vi "Main.vi"() -> ()   [LabVIEW 2018, in "Tracks Repair.lvlib"]
doc: "This template is based off of the Queued Message Handler design pattern and the Queued Message Handler project template that ships with LabVIEW.\n\nThe main difference is that the queue is private to this module and communication between modules is performed via Broadcast and Request events.\n\nRequest events are wrapped in public API methods and are handled in the Event Handling Loop (EHL) of this VI. Any module can register for Broadcast events sent by this module. The EHL generates messages based on user interface actions.\n\nThe Message Handling Loop (MHL) processes messages generated by the EHL, or by other messages. The messages are string values, so new messages can be added easily to the Message Cases case structure in the MHL. Each message cluster can also provide an optional value for Message Data, which is a variant that can be converted to whatever message-specific data is required.\n_____\nBased on Delacor QMH Project Template 4.2.1.64."
uses:
  Tracks Repair.lvlib
  <vilib>/Delacor/Delacor QMH/Libraries/Module Admin_class/Delacor_lib_QMH_Module Admin.lvclass
  SubVi's/Controls/CTL_Basic_cage_settings.ctl
  SubVi's/Controls/CTL_Filter_selector.ctl
  SubVi's/Controls/CTL_Cage_radial_segmentation.ctl
  Module Data--cluster.ctl
  Private API/Data.lvclass
  <vilib>/Delacor/Delacor QMH/Libraries/Message Queue_class/Delacor_lib_QMH_Message Queue.lvclass/Delacor_lib_QMH_Message Queue.ctl
  Stop Argument--cluster.ctl
  <vilib>/Delacor/Delacor QMH/Libraries/Module Admin_class/Delacor_lib_QMH_Module Admin.lvclass/Delacor_lib_QMH_Module Admin.ctl
  Private API/Arguments/Open folder Argument--cluster.ctl
  Private API/Arguments/Load filelist Argument--cluster.ctl
  Private API/Arguments/Preprocess filelist Argument--cluster.ctl
  Show list of files Argument--cluster.ctl
  Show Specific Track Argument--cluster.ctl
  <vilib>/Utility/miscctls.llb/LVPointTypeDef.ctl
  Private API/Data.lvclass/Data.ctl
  <vilib>/Utility/sysdir.llb/System Directory Type.ctl
  SubVi's/Controls/CTL_Post-processing_params.ctl
  SubVi's/Controls/CTL_Mouse_Draw_Params.ctl
  <vilib>/vision/Image Controls.llb/IMAQ Image.ctl
  SubVi's/Controls/CTL_Calibration_parameters.ctl
  SubVi's/Controls/CTL_Dispenser_calibration_info.ctl
  SubVi's/Controls/CTL_Pixel_to_Zone_array.ctl
  <vilib>/Delacor/Delacor QMH/Libraries/Message Queue_class/Delacor_lib_QMH_Enqueue Message (Single).vi
  <vilib>/Delacor/Delacor QMH/Libraries/Module Admin_class/Delacor_lib_QMH_Get External Launch.vi
  Private API/Methods/Write Status.vi
  Private API/Methods/Write Directory path.vi
  Private API/Methods/Write TDMS files paths.vi
  Private API/Methods/Read Directory path.vi
  Private API/Methods/Read TDMS files paths.vi
  <vilib>/Utility/error.llb/Error Cluster From Error Code.vi
  <userlib>/_OpenG.lib/file/file.llb/File Exists - Scalar__ogtk.vi
  <vilib>/ErrorRing/Error Ring.xnode
  <vilib>/Delacor/Delacor QMH/Libraries/Message Queue_class/Delacor_lib_QMH_Message Queue.lvclass
  Tracker.lvlib
panel:
  in  "Cage radial segmentation":T1={"CENTER"={"Radius, mm CENTER"=30}, "MIDFIELD"={"Radius, mm MIDFIELD"=75, "N segments MIDFIELD"=2, "Starting angle MIDFIELD"=0}, "BORDER"={"N segments BORDER"=4, "Starting angle BORDER"=0}} caption="Segmentation" {"BORDER"."N segments BORDER" min=1 max=12; "MIDFIELD"."N segments MIDFIELD" max=8; "CENTER"."Radius, mm CENTER" min=5 step=1}
  in  "Refresh Button":bool
  in  "Apply to All Button":bool
  in  "Apply Button":bool
  in  "Data filtering":T2={"Filter type"=enum."Savitzky-Golay", "Length"=41, "Order"=3} {"Order" min=3 max=11 step=2; "Length" min=5 max=301 step=2}
  in  "Decimate":bool=TRUE
  in  "Diagram (display)":T3(plugin-control)=refnum
  out "Rec. start (SW)":timestamp format="%<%H:%M:%S%3u %Y.%m.%d>T"
  out "Rec. start (HW)":i32
  in  "Settings":T4={"Vert. offset"=0.0, "Hor. offset"=0.0, "Bridge swap"=FALSE, "Twisted neck"=FALSE, "Cage diam."=325, "Magn.rot."=0, "Acq. speed"=0.0} {"Acq. speed" format="%_5f fps"; "Magn.rot." min=-180 max=180 step=1 format="%.0d°"; "Cage diam." format="%.0u mm"; "Hor. offset" format="%#_1f mm"; "Vert. offset" format="%#_1f mm"}
  in  "Open Button":bool
  in  "List of files":i32(listbox)
  in  "Simulate MHL Error":bool
  in  "Simulate EHL Error":bool
  out "error out":errorcluster
  in  "Module Admin":refnum<class "Delacor_lib_QMH_Module Admin.lvclass">
  out "Status":string
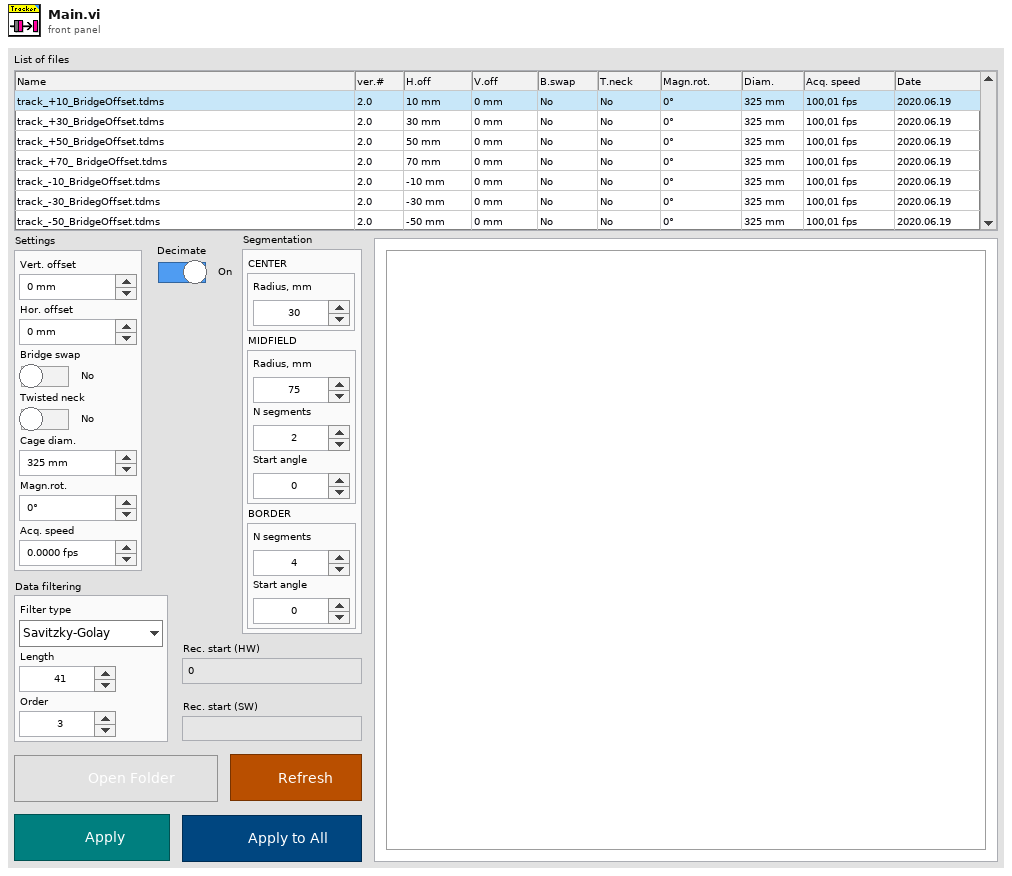
[diagram p1: front panel]
types:
  T1 = typedef "Tracker.lvlib/CTL_Cage_radial_segmentation.ctl" = cluster{"CENTER":cluster{"Radius, mm CENTER":u16}, "MIDFIELD":cluster{"Radius, mm MIDFIELD":u16, "N segments MIDFIELD":u8, "Starting angle MIDFIELD":i16}, "BORDER":cluster{"N segments BORDER":u8, "Starting angle BORDER":i16}}
  T2 = typedef "Tracker.lvlib/CTL_Filter_selector.ctl" = cluster{"Filter type":enum16{"None", "Savitzky-Golay"}, "Length":i32, "Order":i32}
  T3 = typedef "IMAQ Image.ctl" = refnum<image>
  T4 = typedef "Tracker.lvlib/CTL_Basic_cage_settings.ctl" = cluster{"Vert. offset":dbl, "Hor. offset":dbl, "Bridge swap":bool, "Twisted neck":bool, "Cage diam.":i32, "Magn.rot.":i32, "Acq. speed":dbl}
  T5 = typedef "Tracks Repair.lvlib/Module Data--cluster.ctl" = cluster{"Status":string}
  T6 = typedef "Tracks Repair.lvlib/Request Events--cluster.ctl" = cluster{"Stop Module":refnum<user-event>, "Show Panel":refnum<user-event>, "Hide Panel":refnum<user-event>, "Get Module Execution Status":refnum<user-event>, "Show Diagram":refnum<user-event>, "Open folder":refnum<user-event>, "Load filelist":refnum<user-event>, "Preprocess filelist":refnum<user-event>, "Show list of files":refnum<user-event>, "Show Specific Track":refnum<user-event>}
  T7 = enum32{"invalid lock state", "Not Locked", "Locked (No Password)", "Password-protected"}
  T8 = typedef "Tracks Repair.lvlib/Stop Argument--cluster.ctl" = cluster{"Origin":string, "Exit via Stop Module Req?":bool, "Wait for Module to stop?":bool}
  T9 = typedef "Tracks Repair.lvlib/Open folder Argument--cluster.ctl" = cluster{"Open":bool}
  T10 = typedef "Tracks Repair.lvlib/Load filelist Argument--cluster.ctl" = cluster{"Boolean":bool}
  T11 = typedef "Tracks Repair.lvlib/Preprocess filelist Argument--cluster.ctl" = cluster{"Boolean":bool}
  T12 = typedef "Tracks Repair.lvlib/Show list of files Argument--cluster.ctl" = cluster{"Boolean":bool}
  T13 = typedef "Tracks Repair.lvlib/Show Specific Track Argument--cluster.ctl" = cluster{"Track #":i32}
  T14 = typedef "LVPointTypeDef.ctl" = cluster{"Horizontal":i16, "Vertical":i16}
  T15 = enum32{"Invalid", "Standard", "Closed", "Hidden", "Minimized", "Maximized"}
  T16 = typedef "Tracker.lvlib/CTL_Post-processing_params.ctl" = cluster{"Defragment TDMS? (F)":bool, "Start time (SW)":timestamp, "Start time (HW)":u32, "Data filtering":T2, "Mouse drawing parameters":T17, "Size of the image (480x480)":cluster{"Numeric Control":dbl, "Numeric Control":dbl}, "Image ref. in":T3, "Calibration parameters":T18, "Pixel to zone":T20}
  T17 = typedef "Tracker.lvlib/CTL_Mouse_Draw_Params.ctl" = cluster{"Trace length, samples":u16, "Rainbow track":bool, "Rainbow track is speed":bool, "Bright mouse lineout":bool, "Colors array":u32[], "Pixels per mm":dbl}
  T18 = typedef "Tracker.lvlib/CTL_Calibration_parameters.ctl" = cluster{"Timing calibration sw/hw":dbl, "True FPS":dbl, "True frame time, s":dbl, "Disp. calibration info":T19}
  T19 = typedef "Tracker.lvlib/CTL_Dispenser_calibration_info.ctl" = cluster{"Channel":u8, "Speed, µl per ms":dbl}[]
  T20 = typedef "Tracker.lvlib/CTL_Pixel_to_Zone_array.ctl" = i8[][]
  T21 = typedef "System Directory Type.ctl" = i32
  T22 = typedef "Tracker.lvlib/CTL_Settings_cluster.ctl" = cluster{"Defaults":cluster{"Default User":dbl, "VISA Resource Name ":string, "Histogram parameters":T23}, "Recording and saving":cluster{"Researcher name":string, "Name prefix":string, "Data post-processing":T2, "Stop at":dbl, "\"Stop at\" enabled":bool, "Default save folder path":path, "Acquisition FPS":T24}, "Geometry":T25, "IO parameters":T26, "Conditions presets array":T27, "Calibration parameters":T18, "Settings loaded OK":bool}
  T23 = typedef "Tracker.lvlib/CTL_Histogram_parameters.ctl" = cluster{"max":dbl, "min":dbl, "# bins":i32, "threshold":dbl, "thr. type":enum16{"higher accepted", "lower accepted"}}
  T24 = typedef "Tracker.lvlib/CTL_Acquisition_speed_selector.ctl" = enum16{"Max", "Optimal", "Eco"}
  T25 = typedef "Tracker.lvlib/CTL_Segmented_plot_parameters.ctl" = cluster{"Cage diameter, mm":u16, "Starting angle MIDFIELD":i16, "Starting angle BORDER":i16, "Radius, mm CENTER":u16, "Radius, mm MIDFIELD":u16, "N segments MIDFIELD":u8, "N segments BORDER":u8, "R-gap, mm":sgl, "Bridge swap":bool, "Bridge H. offset":sgl, "Bridge V. offset":sgl, "Twisted neck":bool, "Alt. magn. orientation":bool, "Sensor board size":enum16{"Small", "Large"}}
  T26 = typedef "Tracker.lvlib/CTL_IO_params_cluster.ctl" = cluster{"IO general config.":u16, "IO 1 configuration":u16, "IO 2 configuration":u16, "IO 3 configuration":u16, "IO 4 configuration":u16, "Activate ext. RS-232":u16, "IO inversion config.":u16, "Sync capability":u8}
  T27 = typedef "Tracker.lvlib/CTL_Conditions_Array.ctl" = T28[]
  T28 = typedef "Tracker.lvlib/CTL_Conditions_Cluster.ctl" = cluster{"Enabled":bool, "Name":string, "Specifier(s)":cluster{"Specifier enabled":bool, "Condition type":T29, "Comparison type":T30, "Value":dbl, "Validity criteria(s)":cluster{"V. check enabled":bool, "Criteria":T31, "Validity value":dbl}[]}[], "Response":T32, "Has been set":bool}
  T29 = typedef "Tracker.lvlib/CTL_Condition_type.ctl" = enum16{"Speed", "Zone", "Angle to wall"}
  T30 = typedef "Tracker.lvlib/CTL_Comparison_type.ctl" = enum16{"Less", "Less or Equal", "Equal", "Greater or Equal", "Greater", "Not Equal"}
  T31 = typedef "Tracker.lvlib/CTL_Validity_check_criteria.ctl" = enum16{"Running bout (seconds)", "Running bout (meters)"}
  T32 = typedef "Tracker.lvlib/CTL_Response_info.ctl" = cluster{"Response type":T33, "TTL port":T34, "TTL pulse length, ms":dbl}
  T33 = typedef "Tracker.lvlib/CTL_Condition_response_type.ctl" = enum16{"None", "Air puff", "Liquid reward"}
  T34 = typedef "Tracker.lvlib/CTL_Reponse_port_info.ctl" = enum16{"Port 1", "Port 2", "Port 3", "Port 4"}
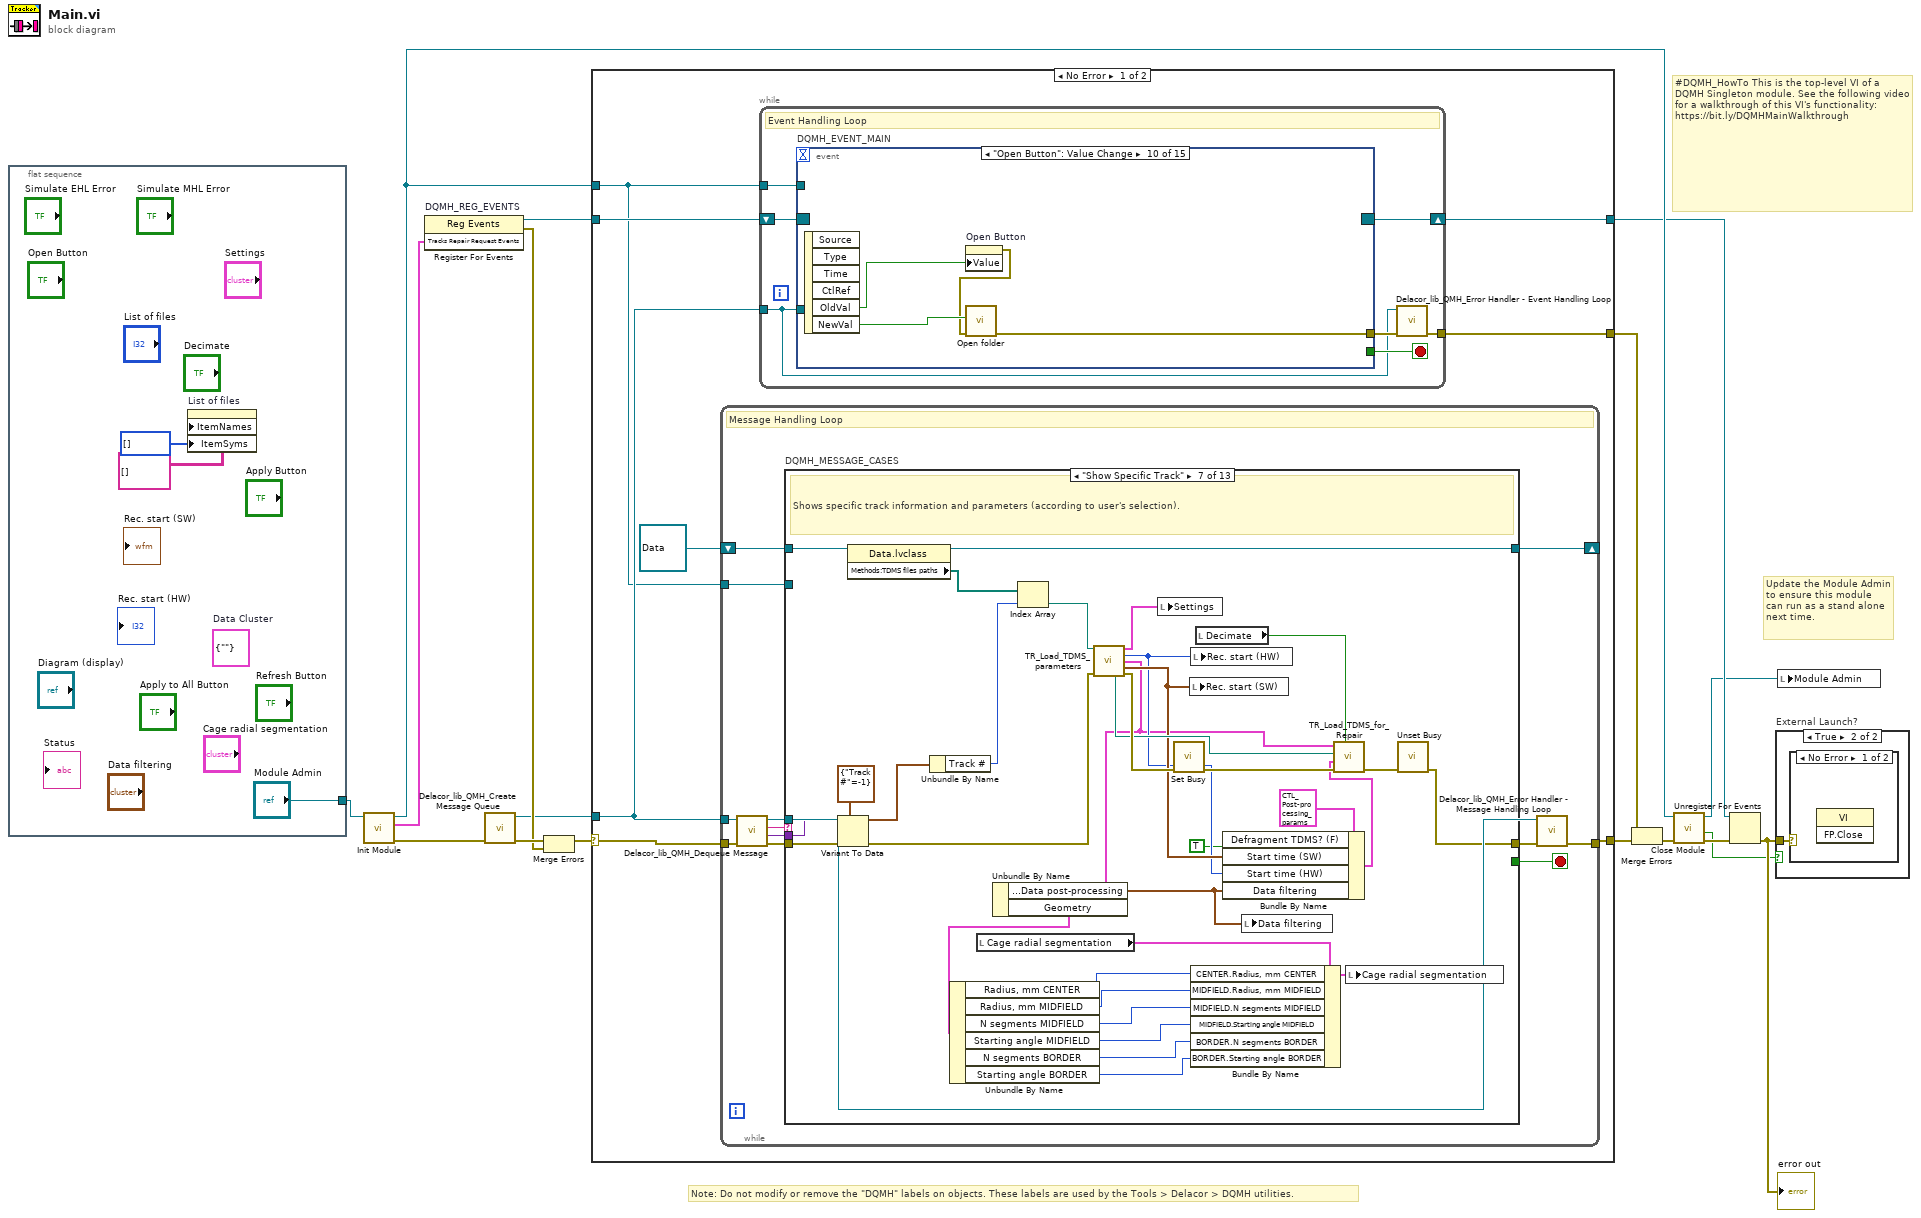
[diagram p0: block diagram]
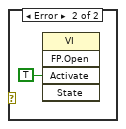
[diagram p3: hidden frame]
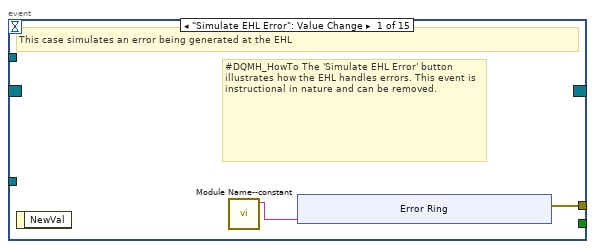
[diagram p4: hidden frame]
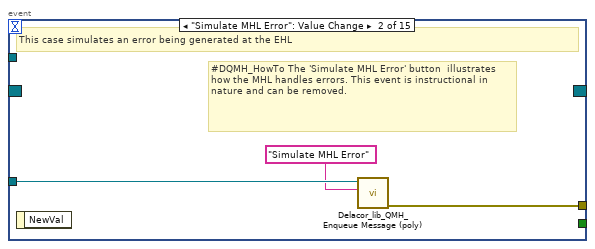
[diagram p5: hidden frame]
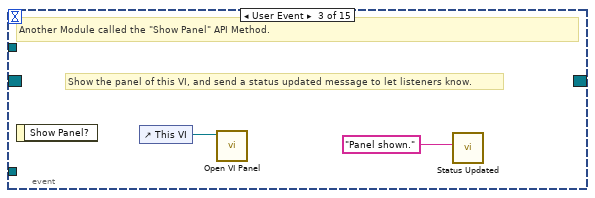
[diagram p6: hidden frame]
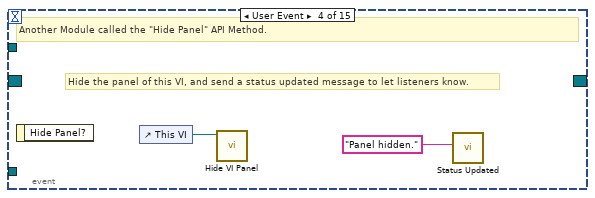
[diagram p7: hidden frame]
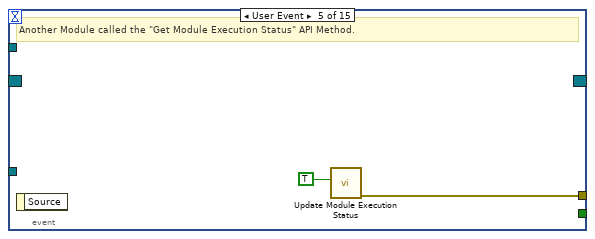
[diagram p8: hidden frame]
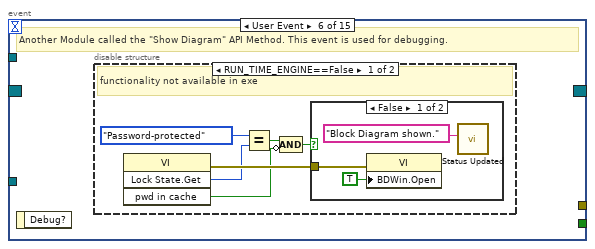
[diagram p9: hidden frame]
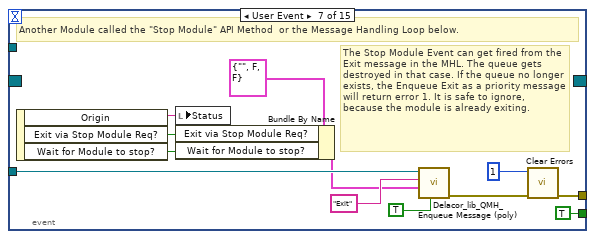
[diagram p12: hidden frame]
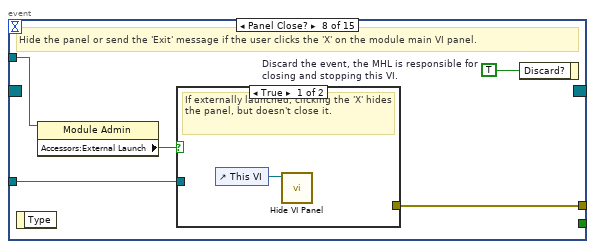
[diagram p13: hidden frame]
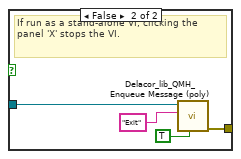
[diagram p14: hidden frame]
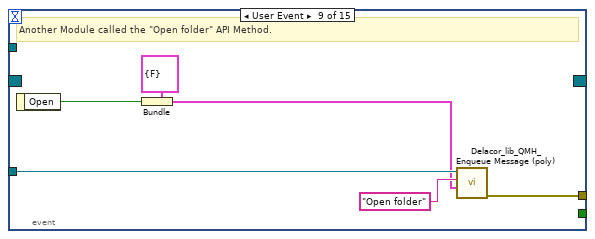
[diagram p15: hidden frame]
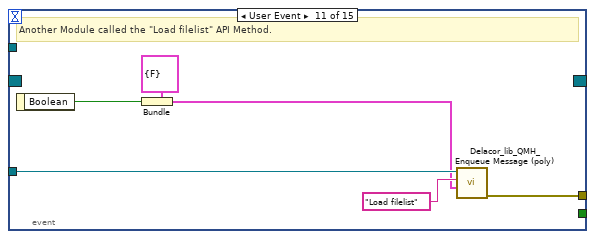
[diagram p16: hidden frame]
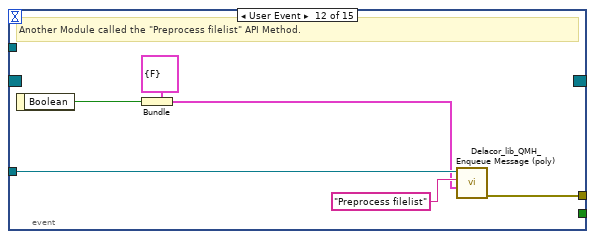
[diagram p17: hidden frame]
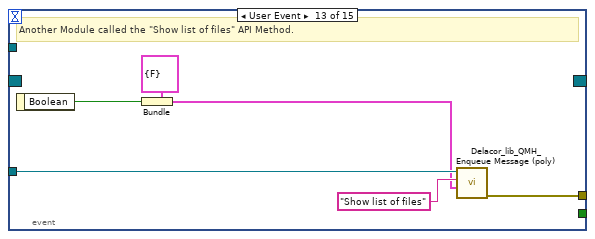
[diagram p18: hidden frame]
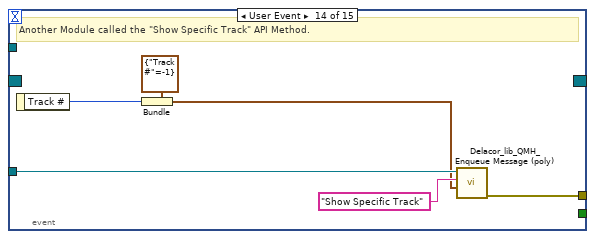
[diagram p19: hidden frame]
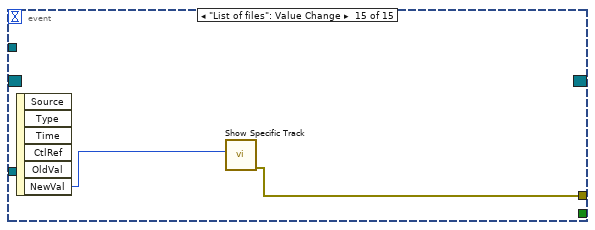
[diagram p20: hidden frame]
diagram:
  # "#DQMH_HowTo This is the top-level VI of a DQMH Singleton module. See the following video for a walkthrough of this VI's functionality: https://bit.ly/DQMHMainWalkthrough"
  # "Note: Do not modify or remove the \"DQMH\" labels on objects. These labels are used by the Tools > Delacor > DQMH utilities."
  # "Update the Module Admin to ensure this module can run as a stand alone next time."
  n1 = flat-sequence {
    tunnel: ["Module Admin"] -> w3
    frame #0 {
      (unwired) T5 {"Status"=""}  # Data Cluster
      n2 = property on="List of files" class="MCListbox (strict)"("ItemNames"=string[][] [] ("Item Names"), "ItemSyms"=i32[] [] ("Item Symbols")) -> ()  [unwired: 2 in, 2 out]
    }
  }
  n3 = call "Init Module.vi"("Singleton Module Admin in"=w3) -> ("error out"=w16:errorcluster, "Tracks Repair Request Events"=w5:T6, "Singleton Module Admin out"=w8:refnum<class "Delacor_lib_QMH_Module Admin.lvclass">)  [unwired: 8 in]
  n4 = register-events "DQMH_REG_EVENTS"(w5) -> (reference out=w6:refnum<event-registration>, error out=w9:errorcluster)  [unwired: 2 in]
  n5 = call <vilib>:"Delacor_lib_QMH_Create Message Queue.vi"("error in (no error)"=w16) -> ("error out"=w11:errorcluster, "Message Queue"=w4:refnum<class "Delacor_lib_QMH_Message Queue.lvclass">)  [unwired: 9 in]
  n6 = Merge Errors(w11, w9) -> (w10:errorcluster)
  n7 = case shown="No Error" w10 {
    selector: w10 -> [w26 w349]
    tunnel: [w28 w349] -> w17
    tunnel: [w25 w346] -> w7
    tunnel: w6 -> [w24 w346]
    tunnel: w4 -> [w23 _]
    tunnel: [w27 _] -> w14
    tunnel: w8 -> [w22 w342]
    frame No Error {
      n8 = while {
        tunnel: w23 -> [w123]
        shift-right: [w127] -> _
        shift-left: refnum<class "Data.lvclass"> refnum ("Tracks Repair.lvlib:Data.lvclass") -> [w128]
        tunnel: w26 -> [w131]
        tunnel: [w129] -> w28
        tunnel: w22 -> [w121]
        stop <- w126 stop-if-true
        # "Message Handling Loop"
        n9 = call-dynamic "Delacor_lib_QMH_Dequeue Message.vi"("error in (no error)"=w131, "Message Queue in"=w123) -> ("error out"=w130:errorcluster, "Message Data"=w124:variant, "Message"=w125:string, "Message Queue out"=w122:refnum<class "Delacor_lib_QMH_Message Queue.lvclass">)  [unwired: 6 in]
        n10 = case "DQMH_MESSAGE_CASES" shown="\"Show Specific Track\"" w125 {
          selector: w125 -> [_ _ _ _ _ _ _ _ _ _ _ _ w329]
          tunnel: w122 -> [_ _ _ _ _ _ _ _ _ _ w297 w319 _]
          tunnel: w130 -> [w150 w154 w170 w193 w218 w244 w277 w280 w282 w287 w304 w325 w331]
          tunnel: [w148 w154 w155 w183 w206 w232 w267 w279 w282 w286 w300 w322 w332] -> w132
          tunnel: w128 -> [w135 w153 w167 w192 w217 w241 w276 w278 w281 w284 w299 w318 w330]
          tunnel: [w134 w153 w166 w185 w208 w240 w272 w278 w281 w284 w299 w318 w327] -> w127
          tunnel: [_ _ _ _ _ _ _ _ _ _ _ w317 _] -> w126
          tunnel: w124 -> [_ _ _ w191 w216 w243 w275 _ _ _ w298 w316 _]
          tunnel: w121 -> [w140 _ _ _ _ _ _ _ _ _ w296 w311 _]
          frame "Initialize" {
            # "#CodeNeeded - Initialize the appearance of the front panel."
            # "#CodeNeeded - Initialize your state data here."
            # "Initialize - Any operation that needs to be done before the module can receive messages. Synchronize Caller Events.vi will inform Start Module.vi that the module has launched and is ready to receive messages. Module Did Init.vi will broadcast that the module initialized."
            n11 = call "Synchronize Caller Events.vi"("error in (no error)"=w150, "Singleton Module Admin in"=w140) -> ("error out"=w149:errorcluster, "Singleton Module Admin out"=w137:refnum<class "Delacor_lib_QMH_Module Admin.lvclass">)  [unwired: 8 in]
            n12 = property class="Module Admin"(reference=w137) -> ("Accessors:External Launch"=w144:bool)  [unwired: 1 in, 2 out]
            n13 = Select(t=T15."Hidden" ("State"), s=w144, f=T15."Standard" ("State")) -> (s? t:f=w141:T15)
            n14 = call "Module Name--constant.vi"() -> ("Module Name"=w147:string)  [unwired: 11 in]
            n15 = property class="VI"("Front Panel.Title"=w147) -> (reference out=w146:refnum<vi>, error out=w152:errorcluster)  [unwired: 2 in]
            n16 = call "Module Name--constant.vi"() -> ("Module Name"=w138:string)  [unwired: 11 in]
            n17 = invoke class="VI" method="FP.Open"(reference=w146, error in=w152, "State"=w141) -> (reference out=w145:refnum<vi>, error out=w151:errorcluster)  [unwired: 2 in, 3 out]
            n18 = property class="Data.lvclass"(reference=w135, "Methods:Status"="Initial Message" ("Initial Message")) -> (reference out=w134:refnum<class "Data.lvclass">)  [unwired: 1 in, 1 out]
            n19 = call "Module Did Init.vi"("error in (no error)"=w149, "Initialized?"=TRUE, "Origin"=w138) -> ("error out"=w148:errorcluster)  [unwired: 8 in]
            n20 = invoke class="VI" method="FP.Center"(reference=w145, error in=w151) -> ()  [unwired: 1 in, 3 out]
            n21 = property on="Pane" class="Pane"("Origin"=T14 {"Horizontal"=0, "Vertical"=0}) -> ()  [unwired: 2 in, 2 out]
          }
          frame "--- Module Specific ---" {
            # "Separator -- The following cases handle messages specific to this Module."
          }
          frame "Open folder" {
            w171 = T21 2 items=["User Home"=0, "User Desktop"=1, "User Documents"=2, "User Application Data"=3, "User Preferences"=4, "User Temporary"=5, "Public Documents"=6, "Public Application Data"=7, "Public Preferences"=8, "Public Cache"=13, "System Core Libraries"=9, "System Installed Libraries"=10, "Application Files"=11, "Boot Volume Root"=12] ("system directory type")
            # "Pops up a folder open dialog for selection of the folder with files to process."
            n22 = call <vilib>:"Get System Directory.vi"("system directory type"=w171) -> ("system directory"=w172:path)  [unwired: 10 in]
            n23 = call "File Dialog"("start path"=w172, "prompt"="Select folder you want to process (with all subfolders)", "button label"="Open", "error in"=w170) -> ("selected path"=w157:path, "cancelled"=w165:bool, "error out"=w156:errorcluster)  [unwired: 8 in, 1 out]
            n24 = call-poly <userlib>:"File Exists__ogtk.vi"("file path"=w157) -> ("is directory"=w164:bool, "exists"=w163:bool)  [unwired: 6 in]
            n25 = Not(x=w165) -> (.not. x?=w162:bool)
            n26 = Not(x=w156) -> (.not. x?=w161:bool)
            n27 = Compound Arithmetic op=AND(w164, w163, w162, w161) -> (w160:bool)
            n28 = case shown="True" w160 {
              tunnel: ["Directory open failed" "Directory open OK"] -> w159
              tunnel: [path "" w178] -> w158
              tunnel: w157 -> [_ w178]
              tunnel: w156 -> [w173 w177]
              tunnel: [w173 w176] -> w155
              frame False {
              }
              frame True {
                n29 = call "Load filelist.vi"("error in (no error)"=w177) -> ("error out"=w176:errorcluster)  [unwired: 10 in]
              }
            }
            n30 = property class="Data.lvclass"(reference=w167, "Methods:Status"=w159, "Methods:Directory path"=w158) -> (reference out=w166:refnum<class "Data.lvclass">)  [unwired: 1 in, 1 out]
          }
          frame "Load filelist" {
            # "Loads a list of files for initial processing from the selected folder (recursive)."
            n31 = property class="Data.lvclass"(reference=w192) -> (reference out=w189:refnum<class "Data.lvclass">, "Methods:Directory path"=w188:path)  [unwired: 1 in, 1 out]
            n32 = Variant To Data(error in=w193, type=T10 {"Boolean"=FALSE} ("Load filelist Argument"), Variant=w191) -> (error out=w186:errorcluster)  [unwired: 1 out]
            n33 = call <userlib>:"List Directory Recursive__ogtk.vi"("error in (no error)"=w186, "pattern"="*.tdms", "Path"=w188) -> ("error out"=w184:errorcluster, "file paths"=w182:path[])  [unwired: 5 in, 2 out]
            n34 = Array Size(array=w182) -> (size(s)=w181:i32)
            n35 = Greater Than 0?(x=w181) -> (x > 0?=w180:bool)
            n36 = case shown="True" w180 {
              tunnel: w189 -> [w200 w205]
              tunnel: [w199 w204] -> w185
              tunnel: w184 -> [w198 w203]
              tunnel: [w194 w202] -> w183
              tunnel: w182 -> [w197 _]
              frame True {
                n37 = property class="Data.lvclass"(reference=w200, error in=w198, "Methods:TDMS files paths"=w197, "Methods:Status"="List of files loaded OK" ("Status")) -> (reference out=w199:refnum<class "Data.lvclass">, error out=w195:errorcluster)
                n38 = call "Preprocess filelist.vi"("error in (no error)"=w195) -> ("error out"=w194:errorcluster)  [unwired: 10 in]
              }
              frame False {
                n39 = property class="Data.lvclass"(reference=w205, error in=w203, "Methods:Status"="List of files is empty!" ("Status")) -> (reference out=w204:refnum<class "Data.lvclass">, error out=w202:errorcluster)
              }
            }
          }
          frame "Preprocess filelist" {
            # "Go through list of TDMS files and check whether they are correct tracker files and can be loaded."
            n40 = property class="Data.lvclass"(reference=w217) -> (reference out=w211:refnum<class "Data.lvclass">, "Methods:TDMS files paths"=w213:path[])  [unwired: 1 in, 1 out]
            n41 = Variant To Data(error in=w218, type=T11 {"Boolean"=FALSE} ("Preprocess filelist Argument"), Variant=w216) -> (error out=w214:errorcluster)  [unwired: 1 out]
            n42 = call "TR_Check_files_format.vi"("error in (no error)"=w214, "TDMS files paths in"=w213) -> ("error out"=w210:errorcluster, "TDMS files paths out"=w209:path[])  [unwired: 8 in]
            n43 = Array Size(array=w209) -> (size(s)=w212:i32)
            n44 = Greater Than 0?(x=w212) -> (x > 0?=w207:bool)
            n45 = case shown="True" w207 {
              tunnel: w211 -> [w225 w230]
              tunnel: [w224 w229] -> w208
              tunnel: w210 -> [w223 w228]
              tunnel: w209 -> [w222 _]
              tunnel: [w219 w226] -> w206
              frame True {
                n46 = property class="Data.lvclass"(reference=w225, error in=w223, "Methods:TDMS files paths"=w222, "Methods:Status"="List of files filtered OK" ("Status")) -> (reference out=w224:refnum<class "Data.lvclass">, error out=w220:errorcluster)
                n47 = call "Show list of files.vi"("error in (no error)"=w220) -> ("error out"=w219:errorcluster)  [unwired: 10 in]
              }
              frame False {
                n48 = property class="Data.lvclass"(reference=w230, error in=w228, "Methods:Status"="List of files is empty after filtering!" ("Status")) -> (reference out=w229:refnum<class "Data.lvclass">, error out=w226:errorcluster)
              }
            }
          }
          frame "Show list of files" {
            # "Shows list of files in the table."
            n49 = Variant To Data(error in=w244, type=T12 {"Boolean"=FALSE} ("Show list of files Argument"), Variant=w243) -> (error out=w239:errorcluster)  [unwired: 1 out]
            n50 = property class="Data.lvclass"(reference=w241, error in=w239) -> (reference out=w240:refnum<class "Data.lvclass">, error out=w238:errorcluster, "Methods:TDMS files paths"=w237:path[])
            n51 = call "TR_Fill_listbox.vi"("error in (no error)"=w238, "Methods:TDMS files paths"=w237) -> ("error out"=w236:errorcluster, "Listbox symbols IDs"=w234:i32[], "Listbox contents"=w235:string[][])  [unwired: 7 in]
            n52 = property on="List of files" class="MCListbox (strict)"(error in=w236, "ItemNames"=w235, "ItemSyms"=w234) -> (error out=w233:errorcluster)  [unwired: 1 in, 1 out]
            n53 = property on="List of files" class="MCListbox (strict)"(error in=w233, "Val(Sgnl)"=0 ("Value (Signaling)")) -> (error out=w232:errorcluster)  [unwired: 1 in, 1 out]
          }
          frame "Show Specific Track" {
            # "Shows specific track information and parameters (according to user's selection)."
            n54 = Variant To Data(error in=w277, type=T13 {"Track #"=-1} ("Show Specific Track Argument"), Variant=w275) -> (data=w273:T13, error out=w269:errorcluster)
            n55 = property class="Data.lvclass"(reference=w276) -> (reference out=w272:refnum<class "Data.lvclass">, "Methods:TDMS files paths"=w271:path[])  [unwired: 1 in, 1 out]
            n56 = Unbundle By Name(w273) -> ("Track #"=w270:i32)
            n57 = local read "Cage radial segmentation"() -> (w253:T1)
            n58 = Index Array(array=w271, index=w270) -> (element=w264:path)
            n59 = call "TR_Load_TDMS_parameters.vi"("TDMS track path in"=w264, "error in (no error)"=w269) -> ("Basic settings"=w254:T4, "1st frame HW timestamp"=w260:i32, "Full settings"=w258:T22, "1st frame SW timestamp"=w261:timestamp, "TDMS track path out"=w263:path, "error out"=w268:errorcluster)  [unwired: 7 in, 1 out]
            n60 = Unbundle By Name(w258) -> ("Recording and saving.Data post-processing"=w257:T2, "Geometry"=w251:T25)
            n61 = Unbundle By Name(w251) -> ("Radius, mm CENTER"=w250:u16, "Radius, mm MIDFIELD"=w249:u16, "N segments MIDFIELD"=w248:u8, "Starting angle MIDFIELD"=w247:i16, "N segments BORDER"=w246:u8, "Starting angle BORDER"=w245:i16)
            n62 = local write "Settings"(w254) -> ()
            n63 = call <vilib>:"Set Busy.vi"("error in (no error)"=w268) -> ("error out"=w265:errorcluster)  [unwired: 9 in, 1 out]
            n64 = local write "Rec. start (SW)"(w261) -> ()
            n65 = local write "Rec. start (HW)"(w260) -> ()
            n66 = Bundle By Name(cluster=w253, "CENTER.Radius, mm CENTER"=w250, "MIDFIELD.Radius, mm MIDFIELD"=w249, "MIDFIELD.N segments MIDFIELD"=w248, "MIDFIELD.Starting angle MIDFIELD"=w247, "BORDER.N segments BORDER"=w246, "BORDER.Starting angle BORDER"=w245) -> (w252:T1)
            n67 = local read "Decimate"() -> (w255:bool)
            n68 = Bundle By Name(cluster=T16 {"Defragment TDMS? (F)"=FALSE, "Start time (SW)"=timestamp(0 s since 1904-01-01), "Start time (HW)"=0, "Data filtering"={"Filter type"=enum."Savitzky-Golay", "Length"=41, "Order"=3}, "Mouse drawing parameters"={"Trace length, samples"=0, "Rainbow track"=FALSE, "Rainbow track is speed"=FALSE, "Bright mouse lineout"=FALSE, "Colors array"=[], "Pixels per mm"=0.0}, "Size of the image (480x480)"={"Numeric Control"=480.0, "Numeric Control"=480.0}, "Image ref. in"=refnum, "Calibration parameters"={"Timing calibration sw/hw"=1.0, "True FPS"=80.0, "True frame time, s"=0.0125, "Disp. calibration info"=[]}, "Pixel to zone"=[]} ("Processing parameters"), "Defragment TDMS? (F)"=TRUE, "Start time (SW)"=w261, "Start time (HW)"=w260, "Data filtering"=w257) -> (w256:T16)
            n69 = local write "Data filtering"(w257) -> ()
            n70 = call "TR_Load_TDMS_for_Repair.vi"("Decimate?"=w255, "error in (no error)"=w265, "Processing parameters"=w256, "TDMS track"=w263, "Settings cluster"=w258) -> ("error out"=w266:errorcluster)  [unwired: 4 in, 2 out]
            n71 = local write "Cage radial segmentation"(w252) -> ()
            n72 = call <vilib>:"Unset Busy.vi"("error in (no error)"=w266) -> ("error out"=w267:errorcluster)  [unwired: 10 in]
          }
          frame "---Copy This Frame---" {
            # "Duplicate this frame when creating new messages.  Change this comment in the duplicated frame to describe this message."
            n73 = Merge Errors(w280) -> (w279:errorcluster)
          }
          frame "--- Exit and Error Handling---" {
            # "Separator - The following cases handle errors and exit messages."
          }
          frame "Simulate MHL Error" {
            # "#DQMH_HowTo The 'Simulate MHL Error' button  illustrates how the MHL handles errors. This event is instructional in nature and can be removed."
            # "Simulate an error occurring at the MHL"
            n74 = call "Module Name--constant.vi"() -> ("Module Name"=w283:string)  [unwired: 11 in]
            n75 = xnode "Error Ring"("parameter 0"=w283) -> ("error out"=w285:errorcluster)
            n76 = Merge Errors(w287, w285) -> (w286:errorcluster)
          }
          frame "Error" {
            # "#CodeRecommended - If you ever change the name of this \"Error\" message, you'll need to update the name in the Check Loop Error.vi as well."
            # "#CodeRecommended - If the module is running in standalone mode (External Launch = FALSE), this code will pop up an error dialog and call the 'Exit' message if an error occurs. Add more fine-grained error handling here."
            # "Error - Check the error message data and respond accordingly. This message is sent by the \"Error Handler\" VIs at the end of each loop in this application."
            n77 = property class="Module Admin"(reference=w296) -> ("Accessors:External Launch"=w295:bool)  [unwired: 1 in, 2 out]
            n78 = Variant To Data(error in=w304, type=errorcluster {"status"=FALSE, "code"=0, "source"=""} ("error constant"), Variant=w298) -> (data=w305:errorcluster, error out=w302:errorcluster)
            n79 = call "Error Reported.vi"("Error"=w305) -> ()  [unwired: 10 in, 1 out]
            n80 = case shown="False" w295 {
              tunnel: [w310 _] -> w301
              tunnel: w297 -> [w308 _]
              tunnel: w305 -> [w309 _]
              frame False {
                # "If the module is running standalone, then pop up an error dialog and call the \"Exit\" message."
                n81 = call <vilib>:"Simple Error Handler.vi"("error in (no error)"=w309) -> ()  [unwired: 4 in, 5 out]
                n82 = call-poly <vilib>:"Delacor_lib_QMH_Enqueue Message (poly).vi"("Priority Message? (F)"=TRUE, "Message"="Exit", "Message Queue in"=w308) -> ("error out"=w310:errorcluster)  [unwired: 7 in, 1 out]
              }
              frame True {
                # "If the module was launched externally, calling the Error Reported broadcast VI is the only action performed by the \"Error\" message. The module's caller can then process the error appropriately."
              }
            }
            n83 = Merge Errors(w302, w301) -> (w300:errorcluster)
            n84 = local write "error out"(w300) -> ()
          }
          frame "Exit" {
            w315 = 91  # 91: not all Exit messages will have an argument
            w317 = TRUE  # Stop the VI
            # "Release the message queue reference"
            # "#CodeNeeded - Add any required cleanup code here"
            # "Exit - Exit the application."
            n85 = Variant To Data(error in=w325, type=T8 {"Origin"="", "Exit via Stop Module Req?"=FALSE, "Wait for Module to stop?"=FALSE} ("Stop Argument"), Variant=w316) -> (data=w313:T8, error out=w321:errorcluster)
            n86 = call <vilib>:"Clear Errors.vi"("error in (no error)"=w321, "specific error code to clear (0: all)"=w315) -> ("error out"=w324:errorcluster)  [unwired: 4 in, 1 out]
            n87 = control-ref of="This VI"() -> (w312:refnum<vi>)
            n88 = call-dynamic "Delacor_lib_QMH_Release Message Queue.vi"("error in (no error)"=w324, "Message Queue"=w319) -> ("error out"=w323:errorcluster)  [unwired: 9 in]
            n89 = call "Handle Exit.vi"("Stop Argument"=w313, "Admin in"=w311, "VI reference"=w312) -> ("error out"=w320:errorcluster)  [unwired: 7 in, 1 out]
            n90 = Merge Errors(w323, w320) -> (w322:errorcluster)
          }
          frame Default {
            # "'Default' case only runs if there is a message that isn't defined in any of the other cases.  Output a programming error."
            n91 = call "Module Name--constant.vi"() -> ("Module Name"=w328:string)  [unwired: 11 in]
            n92 = xnode "Error Ring"("parameter 0"=w329, "parameter 1"=w328) -> ("error out"=w333:errorcluster)
            n93 = property class="Data.lvclass"(reference=w330, "Methods:Status"="Something falled into default case" ("Status")) -> (reference out=w327:refnum<class "Data.lvclass">)  [unwired: 1 in, 1 out]
            n94 = Merge Errors(w331, w333) -> (w332:errorcluster)
          }
        }
        n95 = call-dynamic "Delacor_lib_QMH_Error Handler - Message Handling Loop.vi"("error in (no error)"=w132, "Message Queue in"=w122) -> ("dup error in"=w129:errorcluster)  [unwired: 8 in, 1 out]
      }
      n96 = while {
        tunnel: w23 -> [w29]
        shift-right: [w32] -> w25
        shift-left: w24 -> [w33]
        tunnel: [w34] -> w27
        tunnel: w22 -> [w30]
        stop <- w31 stop-if-true
        # "Event Handling Loop"
        n97 = event "DQMH_EVENT_MAIN" shown="[9] \"Open Button\": Value Change" {
          selector: w33 -> [_ _ _ _ _ _ _ _ _ _ _ _ _ _ _]
          dyn-events: [_ _ _ _ _ _ _ _ _ _ _ _ _ _ _] -> w32
          timeout: _ -> [_ _ _ _ _ _ _ _ _ _ _ _ _ _ _]
          tunnel: [_ _ _ _ _ _ TRUE ("Discard?") _ _ _ _ _ _ _ _] -> w31
          tunnel: w29 -> [_ w46 _ _ _ _ w70 w77 w90 _ w100 w106 w112 w118 _]
          tunnel: [w37 w47 _ _ w53 _ w73 w79 w85 w93 w95 w101 w107 w113 w119] -> w35
          tunnel: w30 -> [_ _ _ _ _ _ _ w76 _ _ _ _ _ _ _]
          event "Simulate EHL Error": Value Change {
            # "#DQMH_HowTo The 'Simulate EHL Error' button  illustrates how the EHL handles errors. This event is instructional in nature and can be removed."
            # "This case simulates an error being generated at the EHL"
            n98 = event-data() -> ()  [unwired: 1 in, 1 out]
            n99 = call "Module Name--constant.vi"() -> ("Module Name"=w36:string)  [unwired: 11 in]
            n100 = xnode "Error Ring"("parameter 0"=w36) -> ("error out"=w37:errorcluster)
          }
          event "Simulate MHL Error": Value Change {
            # "#DQMH_HowTo The 'Simulate MHL Error' button  illustrates how the MHL handles errors. This event is instructional in nature and can be removed."
            # "This case simulates an error being generated at the EHL"
            n101 = event-data() -> ()  [unwired: 1 in, 1 out]
            n102 = call-poly <vilib>:"Delacor_lib_QMH_Enqueue Message (poly).vi"("Message"="Simulate MHL Error", "Message Queue in"=w46) -> ("error out"=w47:errorcluster)  [unwired: 8 in, 1 out]
          }
          event User Event {
            # "Show the panel of this VI, and send a status updated message to let listeners know."
            # "Another Module called the \"Show Panel\" API Method."
            n103 = event-data() -> ()  [unwired: 1 in, 1 out]
            n104 = control-ref of="This VI"() -> (w49:refnum<vi>)
            n105 = call "Open VI Panel.vi"("VI"=w49) -> ()  [unwired: 10 in, 1 out]
            n106 = call "Status Updated.vi"("Status"="Panel shown." ("format string")) -> ()  [unwired: 10 in, 1 out]
          }
          event User Event {
            # "Hide the panel of this VI, and send a status updated message to let listeners know."
            # "Another Module called the \"Hide Panel\" API Method."
            n107 = event-data() -> ()  [unwired: 1 in, 1 out]
            n108 = control-ref of="This VI"() -> (w51:refnum<vi>)
            n109 = call "Hide VI Panel.vi"("VI"=w51) -> ()  [unwired: 10 in, 1 out]
            n110 = call "Status Updated.vi"("Status"="Panel hidden." ("format string")) -> ()  [unwired: 10 in, 1 out]
          }
          event User Event {
            # "Another Module called the \"Get Module Execution Status\" API Method."
            n111 = event-data() -> ()  [unwired: 1 in, 1 out]
            n112 = call "Update Module Execution Status.vi"("Running?"=TRUE) -> ("error out"=w53:errorcluster)  [unwired: 10 in]
          }
          event User Event {
            # "Another Module called the \"Show Diagram\" API Method. This event is used for debugging."
            n113 = event-data() -> ()  [unwired: 1 in, 1 out]
            n114 = disable-structure shown="RUN_TIME_ENGINE==False" {
              frame condition #0 (active) {
                # "functionality not available in exe"
                n115 = invoke class="VI" method="Lock State.Get"() -> (error out=w59:errorcluster, "Get Lock State"=w58:T7, "pwd in cache"=w55:bool)  [unwired: 4 in, 1 out]
                n116 = Equal?(x=T7."Password-protected", y=w58) -> (x = y?=w56:bool)
                n117 = Compound Arithmetic op=AND(w56, invert w55) -> (w54:bool)
                n118 = case shown="False" w54 {
                  tunnel: w59 -> [w62 _]
                  frame False {
                    n119 = property class="VI"(error in=w62, "BDWin.Open"=TRUE ("Block Diagram Window:Open")) -> ()  [unwired: 1 in, 2 out]
                    n120 = call "Status Updated.vi"("Status"="Block Diagram shown." ("format string")) -> ()  [unwired: 10 in, 1 out]
                  }
                  frame True {
                    # "Password-protected VI, and the password is not in the cache. Do not show the diagram."
                  }
                }
              }
              frame condition #1 {
              }
            }
          }
          event User Event {
            # "The Stop Module Event can get fired from the Exit message in the MHL. The queue gets destroyed in that case. If the queue no longer exists, the Enqueue Exit as a priority message will return error 1. It is safe to ignore, because the module is already exiting."
            # "Another Module called the \"Stop Module\" API Method  or the Message Handling Loop below."
            n121 = event-data() -> ("Origin"=w69:string, "Exit via Stop Module Req?"=w65:bool, "Wait for Module to stop?"=w64:bool)  [unwired: 1 in]
            n122 = local write "Status"(w69) -> ()
            n123 = Bundle By Name(cluster=T8 {"Origin"="", "Exit via Stop Module Req?"=FALSE, "Wait for Module to stop?"=FALSE} ("Stop Argument"), "Exit via Stop Module Req?"=w65, "Wait for Module to stop?"=w64) -> (w63:T8)
            n124 = call-poly <vilib>:"Delacor_lib_QMH_Enqueue Message (poly).vi"("Priority Message? (F)"=TRUE, "Message Data"=w63, "Message"="Exit", "Message Queue in"=w70) -> ("error out"=w74:errorcluster)  [unwired: 6 in, 1 out]
            n125 = call <vilib>:"Clear Errors.vi"("error in (no error)"=w74, "specific error code to clear (0: all)"=1) -> ("error out"=w73:errorcluster)  [unwired: 4 in, 1 out]
          }
          event Panel Close? {
            w78 = TRUE  # Discard the event, the MHL is responsible for closing and stopping this VI.
            # "Hide the panel or send the 'Exit' message if the user clicks the 'X' on the module main VI panel."
            n126 = event-data() -> ()  [unwired: 1 in, 1 out]
            n127 = property class="Module Admin"(reference=w76) -> ("Accessors:External Launch"=w75:bool)  [unwired: 1 in, 2 out]
            n128 = case shown="True" w75 {
              tunnel: w77 -> [_ w83]
              tunnel: [_ w84] -> w79
              frame True {
                # "If externally launched, clicking the 'X' hides the panel, but doesn't close it."
                n129 = control-ref of="This VI"() -> (w80:refnum<vi>)
                n130 = call "Hide VI Panel.vi"("VI"=w80) -> ()  [unwired: 10 in, 1 out]
              }
              frame False {
                # "If run as a stand-alone VI, clicking the panel 'X' stops the VI."
                n131 = call-poly <vilib>:"Delacor_lib_QMH_Enqueue Message (poly).vi"("Priority Message? (F)"=TRUE, "Message"="Exit", "Message Queue in"=w83) -> ("error out"=w84:errorcluster)  [unwired: 7 in, 1 out]
              }
            }
            n132 = event-data("Discard?"=w78) -> ()  [unwired: 1 in, 1 out]
          }
          event User Event {
            # "Another Module called the \"Open folder\" API Method."
            n133 = event-data() -> ("Open"=w86:bool)  [unwired: 1 in]
            n134 = Bundle(cluster=T9 {"Open"=FALSE} ("Open folder Argument"), "Open"=w86) -> (w87:T9)
            n135 = call-poly <vilib>:"Delacor_lib_QMH_Enqueue Message (poly).vi"("Message Data"=w87, "Message"="Open folder", "Message Queue in"=w90) -> ("error out"=w85:errorcluster)  [unwired: 7 in, 1 out]
          }
          event "Open Button": Value Change {
            n136 = event-data() -> ("OldVal"=w92:bool, "NewVal"=w94:bool)  [unwired: 1 in, 4 out]
            n137 = property on="Open Button" class="Bool (strict)"("Value"=w92) -> (error out=w91:errorcluster)  [unwired: 2 in, 1 out]
            n138 = call "Open folder.vi"("error in (no error)"=w91, "Open"=w94) -> ("error out"=w93:errorcluster)  [unwired: 9 in]
          }
          event User Event {
            # "Another Module called the \"Load filelist\" API Method."
            n139 = event-data() -> ("Boolean"=w96:bool)  [unwired: 1 in]
            n140 = Bundle(cluster=T10 {"Boolean"=FALSE} ("Load filelist Argument"), "Boolean"=w96) -> (w97:T10)
            n141 = call-poly <vilib>:"Delacor_lib_QMH_Enqueue Message (poly).vi"("Message Data"=w97, "Message"="Load filelist", "Message Queue in"=w100) -> ("error out"=w95:errorcluster)  [unwired: 7 in, 1 out]
          }
          event User Event {
            # "Another Module called the \"Preprocess filelist\" API Method."
            n142 = event-data() -> ("Boolean"=w102:bool)  [unwired: 1 in]
            n143 = Bundle(cluster=T11 {"Boolean"=FALSE} ("Preprocess filelist Argument"), "Boolean"=w102) -> (w103:T11)
            n144 = call-poly <vilib>:"Delacor_lib_QMH_Enqueue Message (poly).vi"("Message Data"=w103, "Message"="Preprocess filelist", "Message Queue in"=w106) -> ("error out"=w101:errorcluster)  [unwired: 7 in, 1 out]
          }
          event User Event {
            # "Another Module called the \"Show list of files\" API Method."
            n145 = event-data() -> ("Boolean"=w108:bool)  [unwired: 1 in]
            n146 = Bundle(cluster=T12 {"Boolean"=FALSE} ("Show list of files Argument"), "Boolean"=w108) -> (w109:T12)
            n147 = call-poly <vilib>:"Delacor_lib_QMH_Enqueue Message (poly).vi"("Message Data"=w109, "Message"="Show list of files", "Message Queue in"=w112) -> ("error out"=w107:errorcluster)  [unwired: 7 in, 1 out]
          }
          event User Event {
            # "Another Module called the \"Show Specific Track\" API Method."
            n148 = event-data() -> ("Track #"=w114:i32)  [unwired: 1 in]
            n149 = Bundle(cluster=T13 {"Track #"=-1} ("Show Specific Track Argument"), "Track #"=w114) -> (w115:T13)
            n150 = call-poly <vilib>:"Delacor_lib_QMH_Enqueue Message (poly).vi"("Message Data"=w115, "Message"="Show Specific Track", "Message Queue in"=w118) -> ("error out"=w113:errorcluster)  [unwired: 7 in, 1 out]
          }
          event "List of files": Value Change {
            n151 = event-data() -> ("NewVal"=w120:i32)  [unwired: 1 in, 5 out]
            n152 = call "Show Specific Track.vi"("Track #"=w120) -> ("error out"=w119:errorcluster)  [unwired: 10 in]
          }
        }
        n153 = call-dynamic "Delacor_lib_QMH_Error Handler - Event Handling Loop.vi"("error in (no error)"=w35, "Message Queue in"=w29) -> ("dup error in"=w34:errorcluster)  [unwired: 8 in, 1 out]
      }
    }
    frame Error {
      # "Synchronize Caller Events.vi will inform Start Module.vi that the module has launched and will let the code calling Start Module.vi register for broadcasts and would permit the caller receive the broadcast that an error occurred at launch time."
      n154 = call "Synchronize Caller Events.vi"("Singleton Module Admin in"=w342) -> ("error out"=w347:errorcluster)  [unwired: 9 in, 1 out]
      n155 = call "Module Name--constant.vi"() -> ("Module Name"=w345:string)  [unwired: 11 in]
      n156 = Format Into String(format string="An error occurred during initialization. %s is no longer running.", w345) -> (resulting string=w343:string)  [unwired: 2 in, 1 out]
      n157 = Merge Errors(w349, w347) -> (w348:errorcluster)
      n158 = call "Error Reported.vi"("Additional Information"=w343, "Error"=w348) -> ()  [unwired: 9 in, 1 out]
    }
  }
  n159 = Merge Errors(w14, w17) -> (w13:errorcluster)
  n160 = call "Close Module.vi"("error in (no error)"=w13, "Module Admin in"=w8) -> ("error out"=w15:errorcluster, "External Launch"=w1:bool, "Module Admin out"=w2:refnum<class "Delacor_lib_QMH_Module Admin.lvclass">)  [unwired: 7 in]
  n161 = Unregister For Events(event registration refnum=w7, error in=w15) -> (error out=w12:errorcluster)
  "error out" <- w12
  n162 = case "External Launch?" shown="True" w1 {
    tunnel: w12 -> [_ w350]
    frame False {
    }
    frame True {
      n163 = case shown="No Error" w350 {
        frame No Error {
          n164 = invoke class="VI" method="FP.Close"() -> ()  [unwired: 3 in, 3 out]
        }
        frame Error {
          n165 = invoke class="VI" method="FP.Open"("Activate"=TRUE ("Activate?")) -> ()  [unwired: 4 in, 5 out]
        }
      }
    }
  }
  n166 = local write "Module Admin"(w2) -> ()
